vi "MiscParams.vi"() -> ()   [LabVIEW 2011]
panel:
  in  "IonLaserEnergy":dbl
  in  "HV_D":dbl
  in  "HV_C":dbl
  in  "HV_B":dbl
  in  "HV_A":dbl
  in  "DspLaserEnergy":dbl
  in  "IG_Detector":dbl
  in  "IG_ToF":dbl
  in  "IG_Source":dbl
  in  "Manometer_AtmP":dbl
  in  "Manometer_MKS":dbl
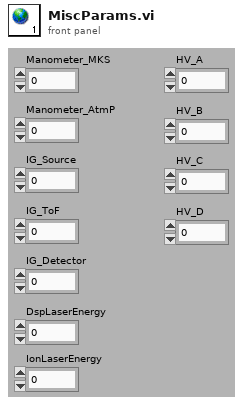
[diagram p1: front panel]
diagram:
